vi "CZE20170723.vi"() -> ()   [LabVIEW 2016]
doc: "DESCRIPTION:\nThis VI simultaneously acquires and generates data on the same board (E-series MIO boards such as the AT-MIO-16E-2). This is a timed signal generation/acquisition, meaning that a hardware clock is used to control the acquisition and update rate for fast and accurate timing. While the output regenerates the same buffer of data, the input is a circular buffered acquisition. This means that a software buffer is used between your DAQ board and LabVIEW. While data is being transferred from your board into one part of the input buffer, LabVIEW is reading data from another part of that buffer. For this reason it is important that you set your acquisition parameters such that LabVIEW reads data out of the buffer fast enough to keep up with the rate at which your board is writing new data into the buffer. If not, unread data will be overwritten and an error will occur.\n\nDue to the fact that E-series MIO type boards have separate clocks dedicated to analog input and analog output, the acquisition and generation can occur at different rates. This example does not synchronize the two clocks.\n\nThis example does synchronize the start of the acquisition and generation using a software trigger. This is accomplished with AO Trigger and Gate Config (an advanced VI) with a trigger source set to \"AI Start Trigger\", which is a signal that will be generated internally when the acquisition begins. No external wiring is required. \n\nINSTRUCTIONS:\n1. Enter the device number, input channels, number of scans to read at a time, scan rate, and input buffer size.\n2. Enter the output channel, the update rate, the output buffer size, and choose the signal to output.\n3. Make the appropriate I/O connections as explained below.\n4. Run the VI.\n\nKEY PARAMETERS:\nThis VI shows how to use the intermediate analog input and analog output DAQ VIs to simultaneously input and output buffered data. On the diagram, notice that AO Start.vi is called before AI Start.vi due to the data dependency of the error cluster. This data dependency causes the acquisition to start after the generation has started.\n\nOn the diagram, notice that the AI Start.vi has a 0 wired for the number of scans to acquire, and the AO Start.vi has a 0 wired for the number of buffer iterations. This sets up continuous acquisition and generation.\n\nThis VI will try to use two DMA channels. If you do not have two available, you can use the Set DAQ Device Information.vi to set the data transfer mode for analog output and/or analog input to use interrupts. \n\nI/O CONNECTIONS:\nConnect to the output and input channels on the I/O connector for your board to match the channels you have chosen on the front panel of this VI.\n\nTo find the actual pin numbers, refer to your hardware user manual.\n\nDAQ VIs USED:\nAI Config.vi, AI Start.vi, AI Read.vi, AI Clear.vi, AO Config.vi, AO Write.vi, AO Trigger and Gate Config.vi, AO Start.vi, AO Clear.vi."
uses:
  <vilib>/Utility/error.llb/DialogType.ctl
  <vilib>/DAQmx/write.llb/DAQmx Write (Analog 1D DBL 1Chan NSamp).vi
  <vilib>/DAQmx/read.llb/DAQmx Read (Analog 2D DBL NChan NSamp).vi
  <vilib>/DAQmx/create/channels.llb/DAQmx Create Channel (AI-Voltage-Basic).vi
  <vilib>/DAQmx/configure/timing.llb/DAQmx Timing (Sample Clock).vi
  <vilib>/DAQmx/create/channels.llb/DAQmx Create Channel (AO-Voltage-Basic).vi
  <vilib>/DAQmx/configure/trigger.llb/DAQmx Start Trigger (Digital Edge).vi
  <vilib>/DAQmx/miscellaneous.llb/DAQmx Fill In Error Info.vi
  <vilib>/Utility/file.llb/Read From Spreadsheet File (DBL).vi
  <resource>/objmgr/daqmx.rc
panel:
  in  "DeviceName":tag="Dev2"
  in  "ケース定数\\n（詳細ヘルプを参照）":bool=TRUE
  in  "DC Volts":dbl=1200.0 min=-10000.0 max=10000.0 step=100.0
  in  "Wfm Type":bool=TRUE
  in  "Abort Load":bool
  in  "HIGH V ON":bool
  out "Time Remaining (sec)":dbl=-6.38378239159465e-16 format="%.1f"
  in  "Load Time (sec)":dbl=2.0 min=0.0 max=10000.0 step=10.0 format="%.1f"
  in  "Load Voltage":dbl=1200.0 min=0.0 max=100000.0 step=100.0
  in  "Load":bool
  out "Num Points":i32=180000
  in  "Duration (min)":dbl=300.0 min=0.0 step=1.0 format="%.1f"
  out "Period (sec)":dbl=0.10000000149011612 format="%.3f"
  in  "Pts/sec":sgl=10.0 min=0 max=10000 step=1 format="%.1f"
  out "Wfm Rate (Hz)":dbl=5.0 format="%.2f"
  out "REV/FWD":dbl=1.0 format="%.2f"
  out "FWD/REV":dbl=1.0 format="%.2f"
  in  "High V/V":dbl=1000.0 min=0.01 max=10000.0 step=100.0 format="%.2f"
  in  "REV Volts":dbl=-200.0 min=-10000.0 max=10000.0 step=100.0
  in  "REV Time (msec)":u32=100 min=1 max=100000 step=1
  in  "FWD Volts":dbl=200.0 min=-10000.0 max=10000.0 step=100.0
  in  "FWD Time (msec)":u32=100 min=1 max=100000 step=1
  out "file name":string
  in  "Read Data":bool
  in  "Start CZE":bool
  in  "Save Data":bool
  out "CZE":cluster{dbl[], dbl[]}(graph)={[0.0, 0.0016666666666666668, 0.0033333333333333335, 0.005, 0.006666666666666667, 0.008333333333333333, 0.01, 0.011666666666666667, 0.013333333333333334, 0.015000000000000001, 0.016666666666666666, 0.018333333333333333, 0.02, 0.021666666666666667, 0.023333333333333334, 0.025, 0.02666666666666667], [0.3002893448067642, 0.29141117530211785, 0.2338674873196842, 0.24110155064381295, 0.1523198704422416, 0.1661303531694248, 0.21249411892116374, 0.21413822415540437, 0.15922511176653875, 0.09674912167511775, 0.12141069594983661, 0.1046408253355316, 0.12864475792492638, 0.11878012798006383, 0.0845827453961778, 0.0655111290069393, 0.07800632588546134]} caption="CV"
  out "timed out?":bool
  in  "stop":bool
  # "DC"
  # "AC"
  # "S\nI\nG\nN\nA\nL\n\nV"
  # "TIME (min)"
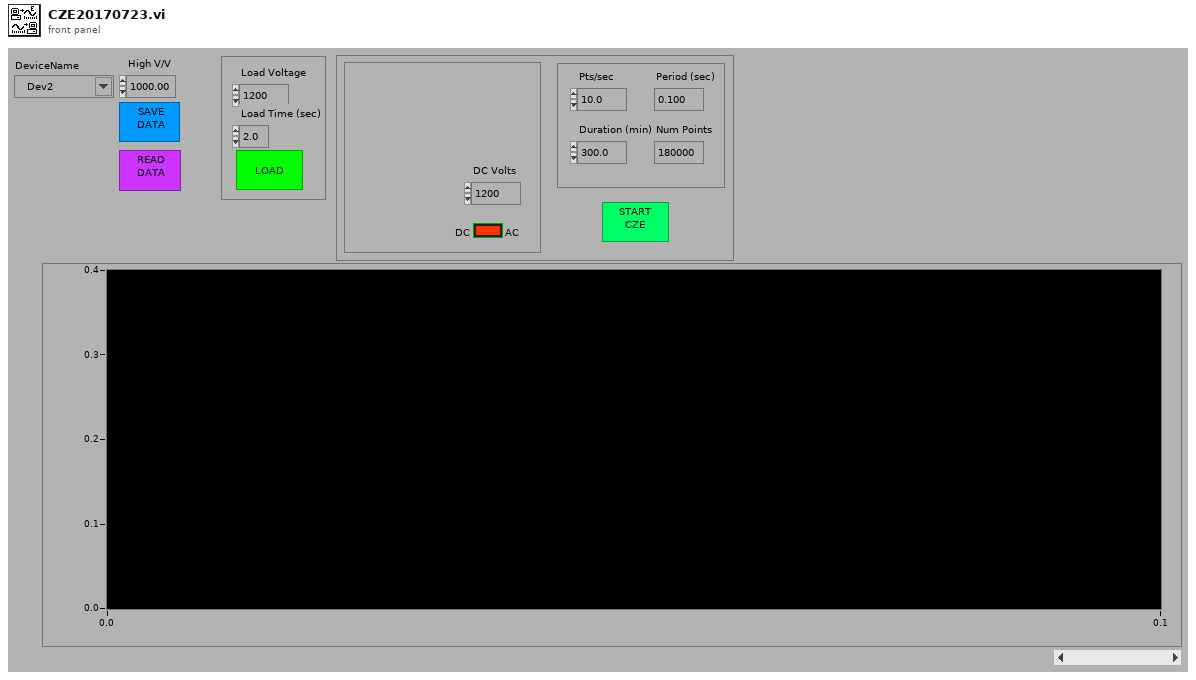
[diagram p1: front panel]
types:
  T1 = cluster{"high limit (0.0)":sgl, "low limit (0.0)":sgl}[]
  T2 = cluster{"coupling (no change:0)":enum16{"no change", "DC", "AC", "GND", "internal ref."}, "input config (no change:0)":enum16{"no change", "differential", "ref. single-ended", "non-ref. single-ended"}}[]
  T3 = enum16{"no change", "none", "trigger on rising edge", "trigger on falling edge", "pause while gate is TTL high", "pause while gate is TTL low"}
  T4 = enum16{"open", "open or create", "create or replace", "create"}
  T5 = typedef "DialogType.ctl" = u16
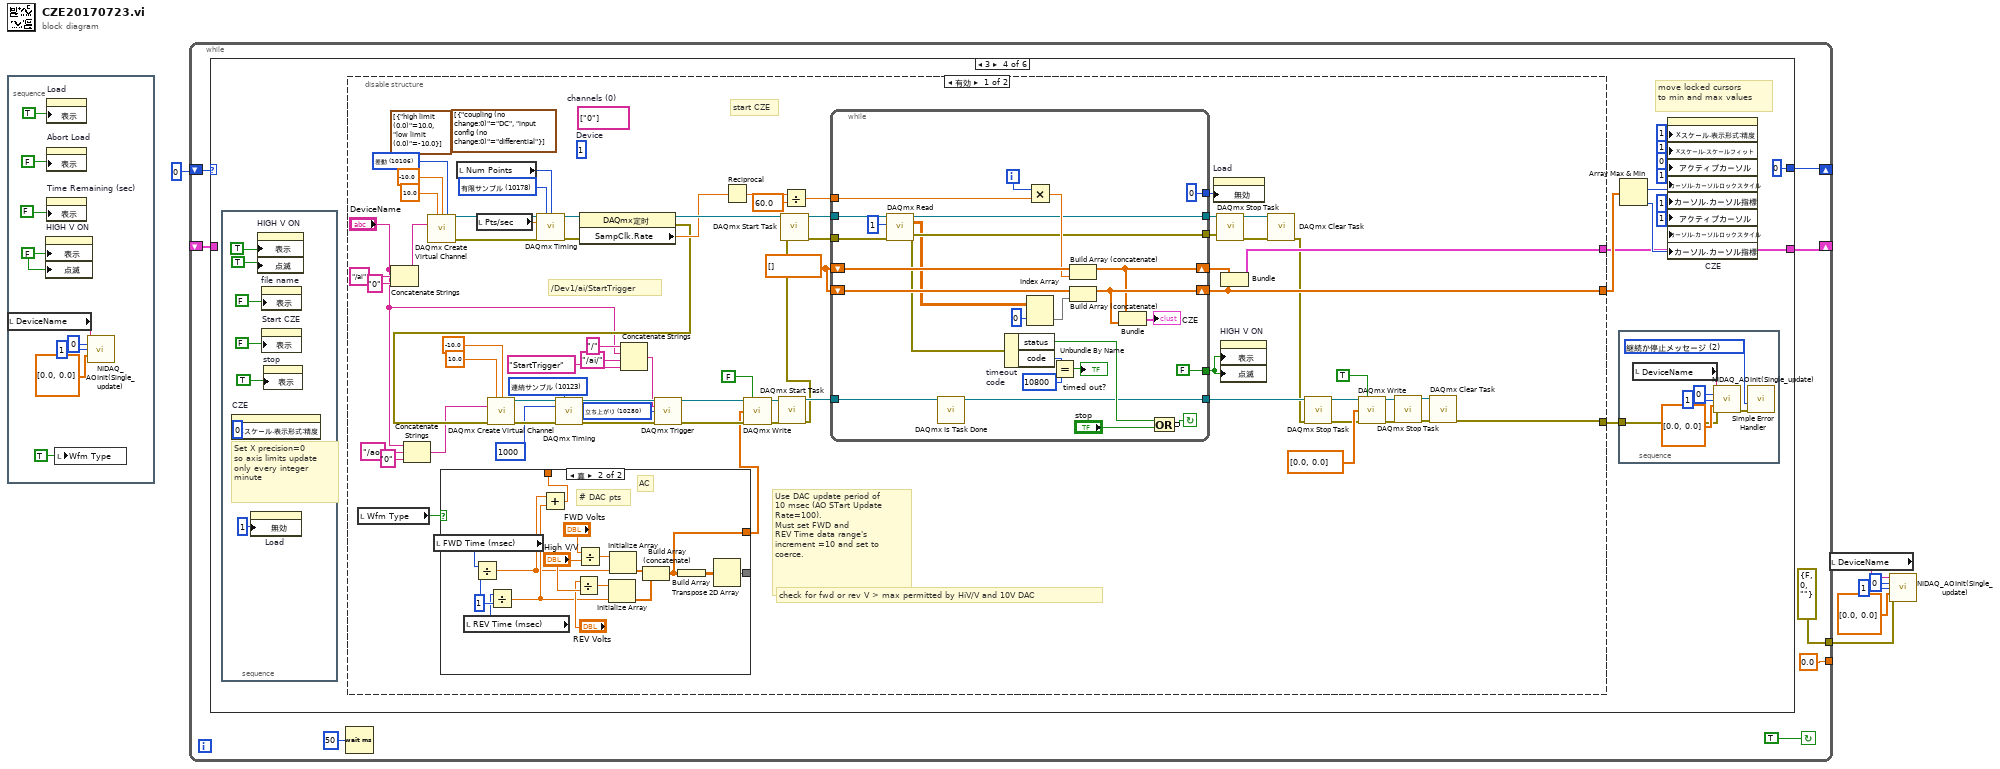
[diagram p0: block diagram]
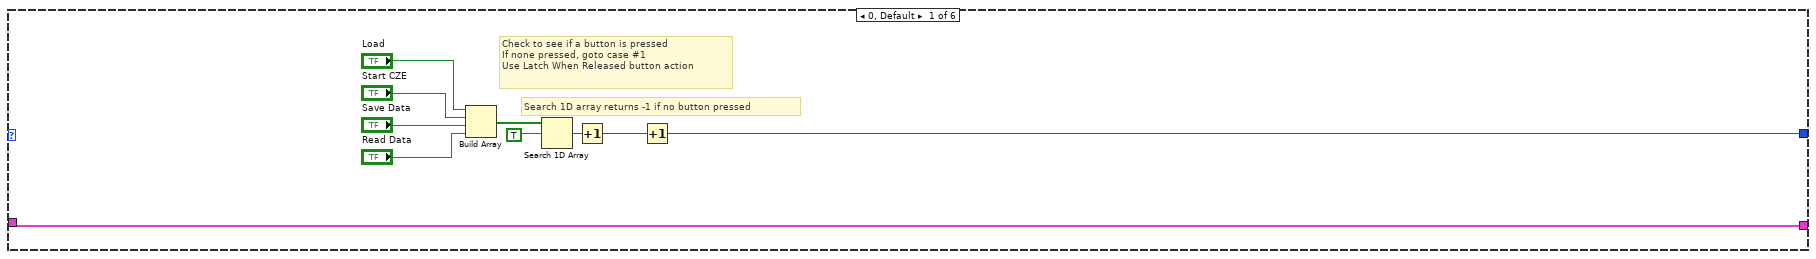
[diagram p2: hidden frame]
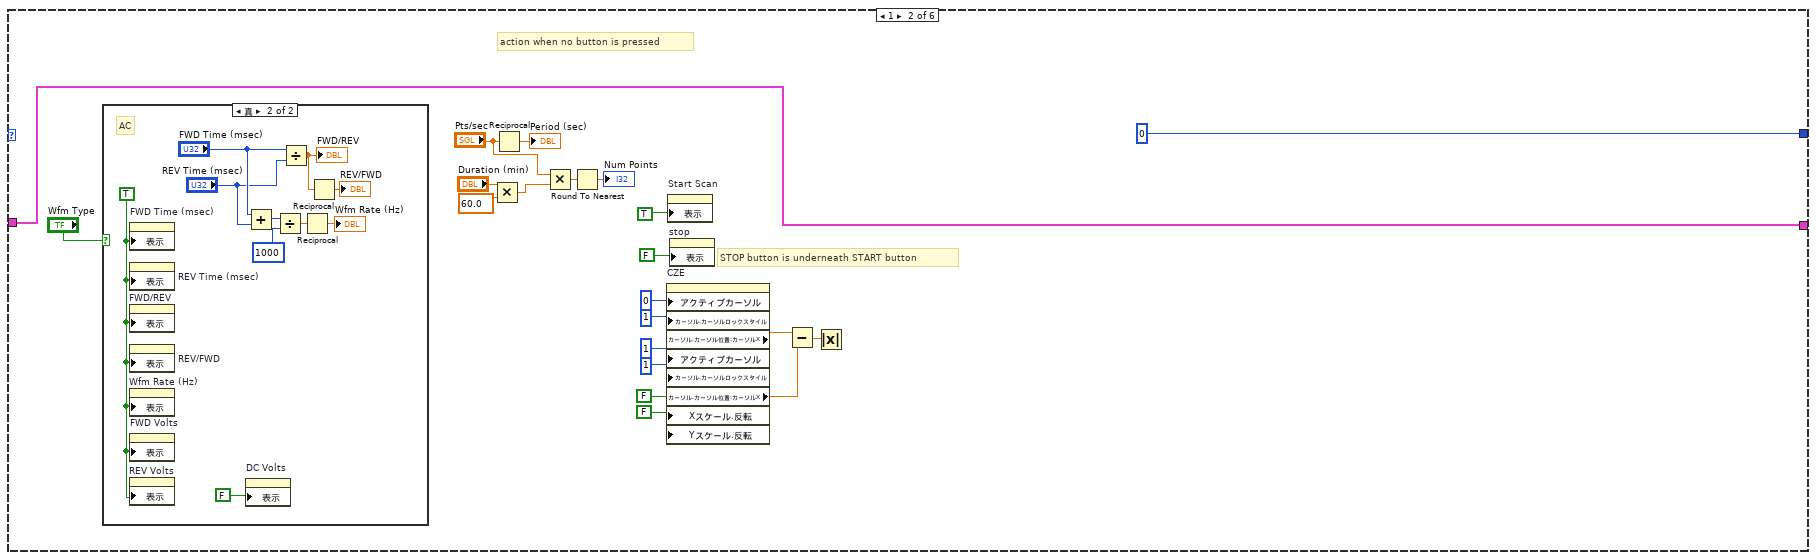
[diagram p3: hidden frame]
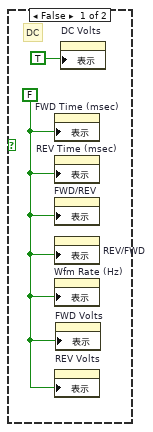
[diagram p4: hidden frame]
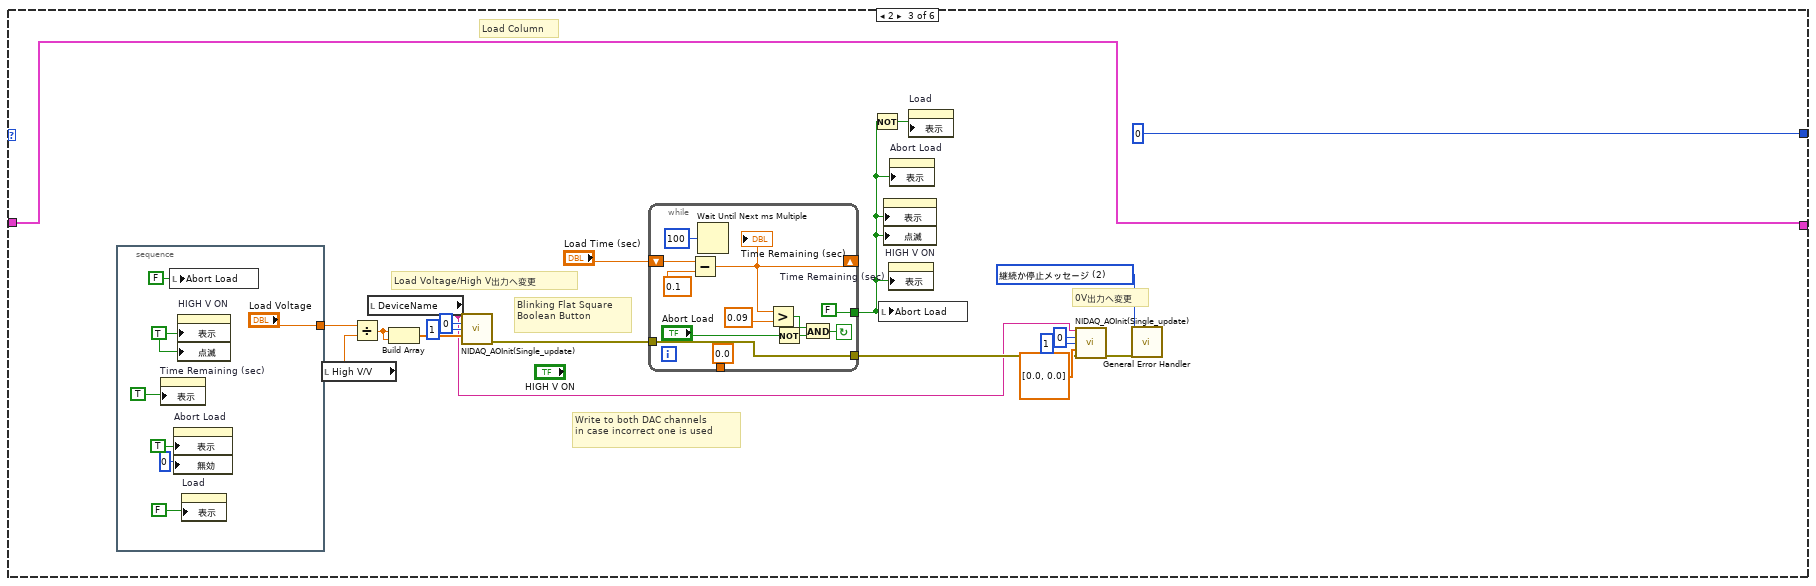
[diagram p5: hidden frame]
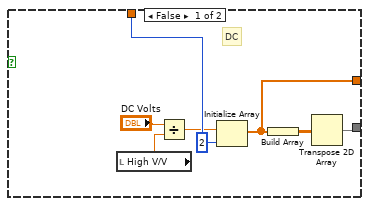
[diagram p6: hidden frame]
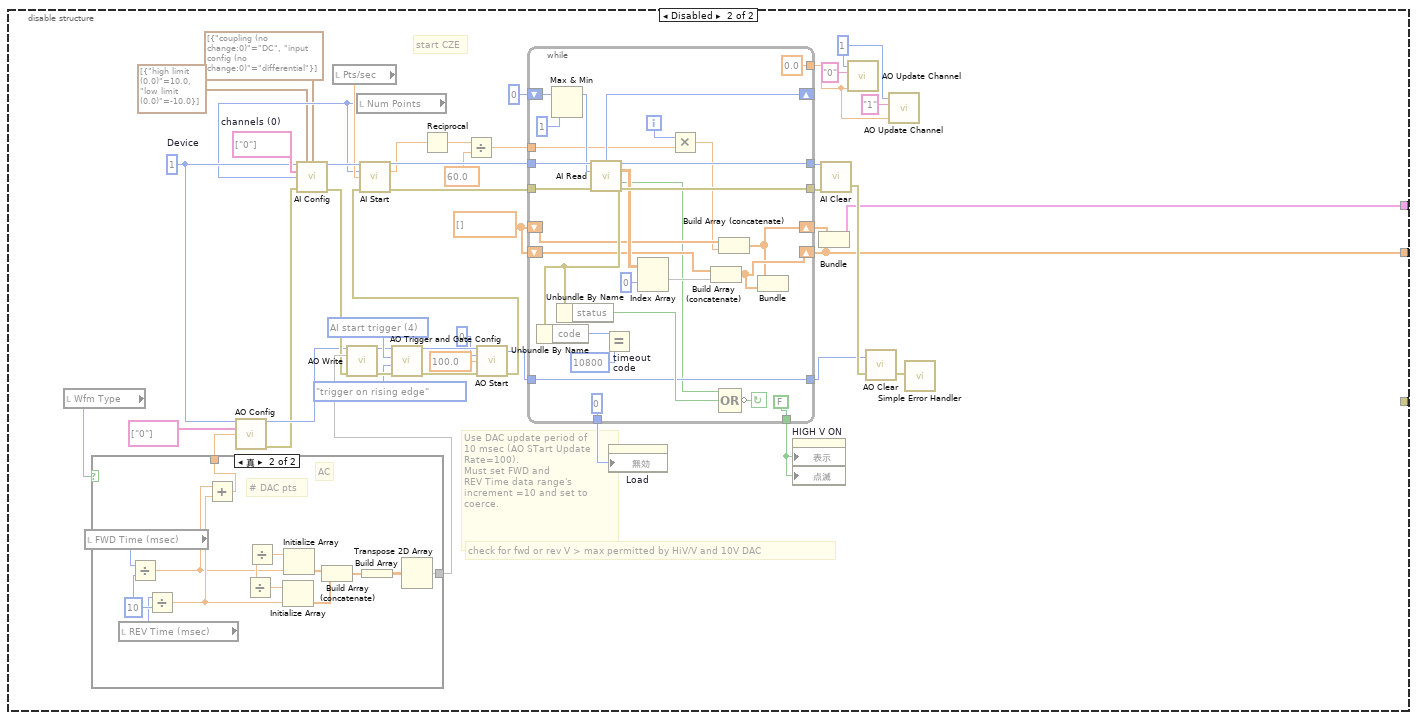
[diagram p7: hidden frame]
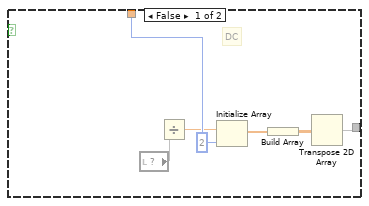
[diagram p8: hidden frame]
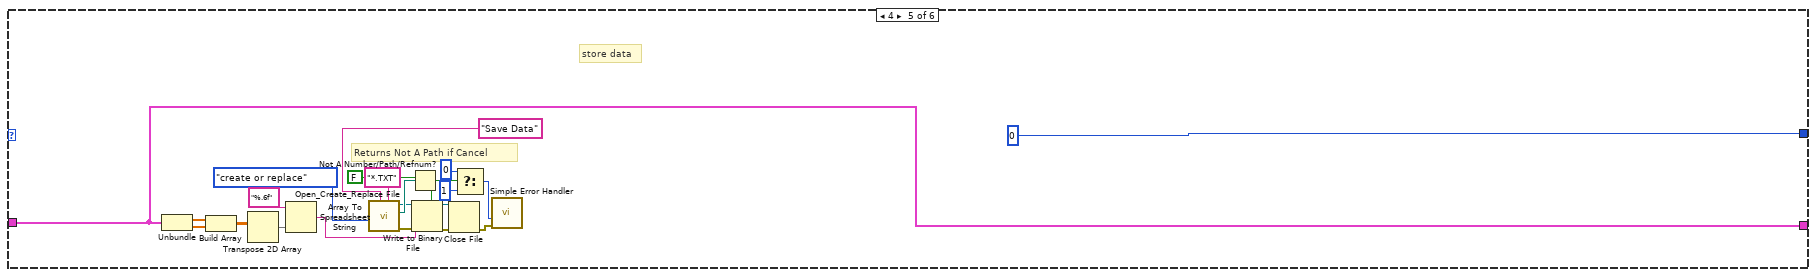
[diagram p9: hidden frame]
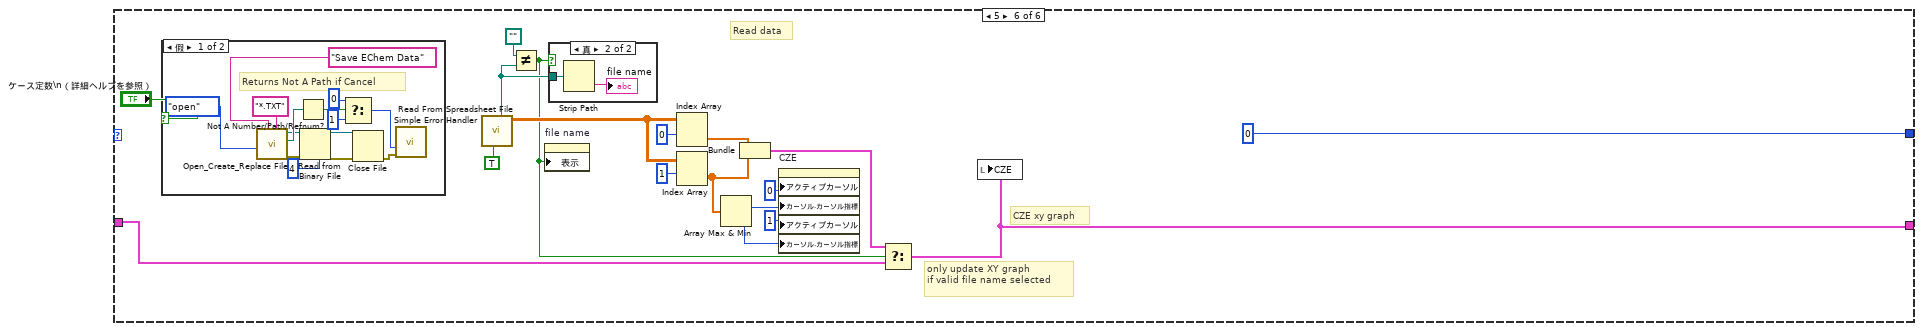
[diagram p10: hidden frame]
diagram:
  n1 = stacked-sequence {
    frame #0 {
      w13 = FALSE ("Visible")
      n2 = local read "DeviceName"() -> (w7:tag)
      n3 = property on="HIGH V ON" class="Bool"("表示"=w13, "点滅"=w13) -> ()  [unwired: 2 in, 2 out]
      n4 = property on="Load" class="Bool"("表示"=TRUE ("Visible")) -> ()  [unwired: 2 in, 2 out]
      n5 = property on="Abort Load" class="Bool (严格)"("表示"=FALSE ("Visible")) -> ()  [unwired: 2 in, 2 out]
      n6 = property on="Time Remaining (sec)" class="DigNum (严格)"("表示"=FALSE ("Visible")) -> ()  [unwired: 2 in, 2 out]
      n7 = local write "Wfm Type"(TRUE ("Wfm Type")) -> ()
      n8 = call "NIDAQ_AOInit(Single_update).vi"("DeviceName"=w7, "CH_A"=0, "CH_B"=1, "Single_point"=dbl[] [0.0, 0.0]) -> ()  [unwired: 11 in, 1 out]
    }
  }
  n9 = while {
    tunnel: [0.0] -> _
    shift-left: _ -> [w20]
    shift-right: [w21] -> _
    shift-left: 0 -> [w23]
    shift-right: [w22] -> _
    tunnel: [errorcluster {"status"=FALSE, "code"=0, "source"=""} ("error in (no error)")] -> w2
    stop <- TRUE continue-if-true
    n10 = case shown="3" w23 {
      tunnel: [w25 0 0 ("t") 0 0 0 ("t")] -> w22
      tunnel: [w28 w44 w83 w108 w348 w368] -> w21
      tunnel: w20 -> [w28 w44 w83 _ w348 w366]
      frame 0, Default {
        # "Check to see if a button is pressed\nIf none pressed, goto case #1\nUse Latch When Released button action"
        # "Search 1D array returns -1 if no button pressed"
        n11 = Build Array("Load", "Start CZE", "Save Data", "Read Data") -> (w31:bool[])
        n12 = Search 1D Array(1D array=w31, element=TRUE) -> (index of element=w29:i32)  [unwired: 1 in]
        n13 = Increment(x=w29) -> (x+1=w27:i32)
        n14 = Increment(x=w27) -> (x+1=w25:i32)
      }
      frame 1 {
        # "STOP button is underneath START button"
        # "action when no button is pressed"
        n15 = case shown="真" "Wfm Type" {
          frame False {
            w55 = FALSE
            # "DC"
            n16 = property on="FWD Time (msec)" class="DigNum (严格)"("表示"=w55) -> ()  [unwired: 2 in, 2 out]
            n17 = property on="REV Time (msec)" class="DigNum (严格)"("表示"=w55) -> ()  [unwired: 2 in, 2 out]
            n18 = property on="FWD/REV" class="DigNum (严格)"("表示"=w55) -> ()  [unwired: 2 in, 2 out]
            n19 = property on="REV/FWD" class="DigNum (严格)"("表示"=w55) -> ()  [unwired: 2 in, 2 out]
            n20 = property on="Wfm Rate (Hz)" class="DigNum (严格)"("表示"=w55) -> ()  [unwired: 2 in, 2 out]
            n21 = property on="REV Volts" class="DigNum (严格)"("表示"=w55) -> ()  [unwired: 2 in, 2 out]
            n22 = property on="FWD Volts" class="DigNum (严格)"("表示"=w55) -> ()  [unwired: 2 in, 2 out]
            n23 = property on="DC Volts" class="DigNum (严格)"("表示"=TRUE ("Visible")) -> ()  [unwired: 2 in, 2 out]
          }
          frame True {
            w58 = TRUE
            # "AC"
            n24 = property on="FWD Time (msec)" class="DigNum (严格)"("表示"=w58) -> ()  [unwired: 2 in, 2 out]
            n25 = property on="REV Time (msec)" class="DigNum (严格)"("表示"=w58) -> ()  [unwired: 2 in, 2 out]
            n26 = property on="FWD/REV" class="DigNum (严格)"("表示"=w58) -> ()  [unwired: 2 in, 2 out]
            n27 = property on="REV/FWD" class="DigNum (严格)"("表示"=w58) -> ()  [unwired: 2 in, 2 out]
            n28 = property on="Wfm Rate (Hz)" class="DigNum (严格)"("表示"=w58) -> ()  [unwired: 2 in, 2 out]
            n29 = property on="FWD Volts" class="DigNum (严格)"("表示"=w58) -> ()  [unwired: 2 in, 2 out]
            n30 = property on="REV Volts" class="DigNum (严格)"("表示"=w58) -> ()  [unwired: 2 in, 2 out]
            n31 = Add(x="FWD Time (msec)", y="REV Time (msec)") -> (x+y=w64:u32)
            n32 = property on="DC Volts" class="DigNum (严格)"("表示"=FALSE ("Visible")) -> ()  [unwired: 2 in, 2 out]
            n33 = Divide(x=w64, y=u32 1000) -> (x/y=w60:dbl)
            n34 = Divide(x="FWD Time (msec)", y="REV Time (msec)") -> (x/y=w66:dbl)
            "FWD/REV" <- w66
            n35 = Reciprocal(x=w60) -> (1/x=→"Wfm Rate (Hz)":dbl)
            n36 = Reciprocal(x=w66) -> (1/x=→"REV/FWD":dbl)
          }
        }
        n37 = Multiply(x="Duration (min)", y=60.0) -> (x*y=w38:dbl)
        n38 = Reciprocal(x="Pts/sec") -> (1/x=→"Period (sec)":sgl)
        n39 = Multiply(x="Pts/sec", y=w38) -> (x*y=w41:dbl)
        n40 = Round To Nearest(number=w41) -> (nearest integer value=→"Num Points":dbl)
        n41 = property on="CZE" class="XYGraph (严格)"("アクティブカーソル"=u32 0 ("Active Cursor"), "カーソル.カーソルロックスタイル"=u32 1 ("Cursor Locked"), "アクティブカーソル"=u32 1 ("Active Cursor"), "カーソル.カーソルロックスタイル"=u32 1 ("Cursor Locked"), "Xスケール.反転"=FALSE ("X Flipped"), "Yスケール.反転"=FALSE ("Y Flipped")) -> ("カーソル.カーソル位置:カーソルX"=w48:dbl, "カーソル.カーソル位置:カーソルX"=w47:dbl)  [unwired: 2 in, 2 out]
        n42 = property on="Start Scan" class="Bool"("表示"=TRUE ("Visible")) -> ()  [unwired: 2 in, 2 out]
        n43 = property on="stop" class="Bool"("表示"=FALSE ("Visible")) -> ()  [unwired: 2 in, 2 out]
        n44 = Subtract(x=w48, y=w47) -> (x-y=w49:dbl)
        n45 = Absolute Value(x=w49) -> ()  [unwired: 1 out]
      }
      frame 2 {
        w67 = T5 2 items=["ダイアログなし", "OKメッセージ", "継続か停止メッセージ", "OKメッセージ+警告", "継続/停止+警告"] ("type of dialog (OK msg:1)")
        # "Load Voltage/High V出力へ変更"
        # "0V出力へ変更"
        # "Blinking Flat Square\nBoolean Button"
        # "Write to both DAC channels\nin case incorrect one is used"
        # "Load Column"
        n46 = stacked-sequence {
          tunnel: ["Load Voltage"] -> w82
          frame #0 {
            w104 = TRUE ("Visible")
            n47 = property on="Time Remaining (sec)" class="DigNum (严格)"("表示"=TRUE ("Visible")) -> ()  [unwired: 2 in, 2 out]
            n48 = local write "Abort Load"(FALSE ("Abort Load")) -> ()
            n49 = property on="Abort Load" class="Bool (严格)"("表示"=TRUE ("Visible"), "無効"=u8 0 ("Disabled")) -> ()  [unwired: 2 in, 2 out]
            n50 = property on="HIGH V ON" class="Bool"("表示"=w104, "点滅"=w104) -> ()  [unwired: 2 in, 2 out]
            n51 = property on="Load" class="Bool"("表示"=FALSE ("Visible")) -> ()  [unwired: 2 in, 2 out]
          }
        }
        n52 = local read "High V/V"() -> (w81:dbl)
        n53 = Divide(x=w82, y=w81) -> (x/y=w73:dbl)
        n54 = local read "DeviceName"() -> (w69:tag)
        n55 = Build Array(w73, w73) -> (w72:dbl[])
        n56 = call "NIDAQ_AOInit(Single_update).vi"("DeviceName"=w69, "CH_A"=0, "CH_B"=1, "Single_point"=w72) -> ("error out"=w71:errorcluster)  [unwired: 11 in]
        n57 = while {
          tunnel: [0.0] -> _
          tunnel: [FALSE] -> w79
          shift-left: "Load Time (sec)" -> [w96]
          shift-right: [w87] -> _
          tunnel: w71 -> [w86]
          tunnel: [w86] -> w70
          stop <- w94 continue-if-true
          n58 = Subtract(x=w96, y=0.1) -> (x-y=w87:dbl)
          "Time Remaining (sec)" <- w87
          n59 = Wait Until Next ms Multiple(millisecond multiple=u32 100) -> ()  [unwired: 1 out]
          n60 = Greater?(x=w87, y=0.09) -> (0:w93:bool)
          n61 = Not(x="Abort Load") -> (.not. x?=w91:bool)
          n62 = And(x=w93, y=w91) -> (x .and. y?=w94:bool)
        }
        n63 = Not(x=w79) -> (.not. x?=w84:bool)
        n64 = local write "Abort Load"(w79) -> ()
        n65 = property on="HIGH V ON" class="Bool"("表示"=w79, "点滅"=w79) -> ()  [unwired: 2 in, 2 out]
        n66 = property on="Time Remaining (sec)" class="DigNum (严格)"("表示"=w79) -> ()  [unwired: 2 in, 2 out]
        n67 = property on="Abort Load" class="Bool (严格)"("表示"=w79) -> ()  [unwired: 2 in, 2 out]
        n68 = property on="Load" class="Bool"("表示"=w84) -> ()  [unwired: 2 in, 2 out]
        n69 = call "NIDAQ_AOInit(Single_update).vi"("DeviceName"=w69, "CH_A"=0, "CH_B"=1, "Single_point"=dbl[] [0.0, 0.0], "error in (no error)"=w70) -> ("error out"=w68:errorcluster)  [unwired: 10 in]
        n70 = call <vilib>:"General Error Handler.vi"("type of dialog (OK msg:1)"=w67, "error in (no error)"=w68) -> ()  [unwired: 9 in, 5 out]
      }
      frame 3 {
        # "move locked cursors\nto min and max values"
        n71 = stacked-sequence {
          frame #0 {
            # "Set X precision=0\nso axis limits update\nonly every integer\nminute"
            n72 = property on="CZE" class="XYGraph (严格)"("Xスケール.表示形式:精度"=u8 0 ("X Precision")) -> ()  [unwired: 2 in, 2 out]
            n73 = property on="Load" class="Bool"("無効"=u8 1 ("Disabled")) -> ()  [unwired: 2 in, 2 out]
            n74 = property on="HIGH V ON" class="Bool"("表示"=TRUE ("Visible"), "点滅"=TRUE ("Blinking")) -> ()  [unwired: 2 in, 2 out]
            n75 = property on="file name" class="Str"("表示"=FALSE ("Visible")) -> ()  [unwired: 2 in, 2 out]
            n76 = property on="Start CZE" class="Bool"("表示"=FALSE ("Visible")) -> ()  [unwired: 2 in, 2 out]
            n77 = property on="stop" class="Bool"("表示"=TRUE ("Visible")) -> ()  [unwired: 2 in, 2 out]
          }
        }
        n78 = disable-structure shown="有効" {
          disable-tunnel: [w191 w263] -> w113
          disable-tunnel: [w189 w261] -> w108
          disable-tunnel: [w126 _] -> w105
          frame Enabled {
            w161 = 10178 items=["有限サンプル"=10178, "連続サンプル"=10123, "ハードウェアタイミングシングルポイント"=12522] ("sample mode")
            w169 = 10106 items=["デフォルト"=-1, "基準化シングルエンド"=10083, "非基準化シングルエンド"=10078, "差動"=10106, "擬似差動"=12529] ("input terminal configuration")
            w170 = 10123 items=["有限サンプル"=10178, "連続サンプル"=10123, "ハードウェアタイミングシングルポイント"=12522] ("sample mode")
            w180 = 10280 items=["立ち上がり"=10280, "立ち下がり"=10171] ("edge")
            (unwired) T1 [{"high limit (0.0)"=10.0, "low limit (0.0)"=-10.0}] ("input limits (no change)")
            (unwired) T2 [{"coupling (no change:0)"=enum."DC", "input config (no change:0)"=enum."differential"}] ("coupling & input config (no change:0)")
            (unwired) i16 1  # Device
            (unwired) string[] ["0"]  # channels (0)
            w188 = sgl[] []
            # "/Dev1/ai/StartTrigger"
            # "Use DAC update period of\n10 msec (AO STart Update\nRate=100).\nMust set FWD and\nREV Time data range's\nincrement =10 and set to\ncoerce."
            # "check for fwd or rev V > max permitted by HiV/V and 10V DAC"
            # "start CZE"
            n79 = local read "Wfm Type"() -> (w182:bool)
            n80 = Concatenate Strings("DeviceName", "/ai", "0" ("文字列")) -> (w147:string)
            n81 = Concatenate Strings("DeviceName", "/ao", "0" ("文字列")) -> (w144:string)
            n82 = call-poly <vilib>:"DAQmx Create Virtual Channel.vi"("maximum value"=10.0, "minimum value"=-10.0, "input terminal configuration"=w169, "physical channels"=w147) -> ("task out"=w156:refnum<k21>, "error out"=w164:errorcluster)  [unwired: 10 in]
            n83 = case shown="真" w182 {
              tunnel: [w224 w240] -> _
              tunnel: [w222 w226] -> _
              tunnel: [w218 w225] -> w135
              frame False {
                w222 = 2
                # "DC"
                n84 = local read "High V/V"() -> (w219:dbl)
                n85 = Divide(x="DC Volts", y=w219) -> (x/y=w221:dbl)
                n86 = Initialize Array(w221, w222) -> (w218:dbl[])
                n87 = Build Array(w218) -> (w223:dbl[][])
                n88 = Transpose 2D Array(2D array=w223) -> (transposed array=w224:dbl[][])
              }
              frame True {
                w234 = u32 1 ("y")
                # "AC"
                # "# DAC pts"
                n89 = local read "FWD Time (msec)"() -> (w232:u32)
                n90 = local read "REV Time (msec)"() -> (w233:u32)
                n91 = Divide(x=w232, y=w234) -> (x/y=w227:dbl)
                n92 = Divide(x=w233, y=w234) -> (x/y=w228:dbl)
                n93 = Add(x=w227, y=w228) -> (x+y=w226:dbl)
                n94 = Divide(x="REV Volts", y="High V/V") -> (x/y=w236:dbl)
                n95 = Divide(x="FWD Volts", y="High V/V") -> (x/y=w237:dbl)
                n96 = Initialize Array(w236, w228) -> (w230:dbl[])
                n97 = Initialize Array(w237, w227) -> (w231:dbl[])
                n98 = Build Array (concatenate)(w231, w230) -> (w225:dbl[])
                n99 = Build Array(w225) -> (w229:dbl[][])
                n100 = Transpose 2D Array(2D array=w229) -> (transposed array=w240:dbl[][])
              }
            }
            n101 = local read "Num Points"() -> (w162:i32)
            n102 = local read "Pts/sec"() -> (w163:sgl)
            n103 = call-poly <vilib>:"DAQmx Timing.vi"("task/channels in"=w156, "sample mode"=w161, "samples per channel"=w162, "rate"=w163, "error in"=w164) -> ("task out"=w160:refnum<k21>, "error out"=w159:errorcluster)  [unwired: 9 in]
            n104 = property class="DAQmx定时"(reference=w160, error in=w159) -> (reference out=w158:refnum<k21>, error out=w154:errorcluster, "SampClk.Rate"=w157:dbl)
            n105 = call-poly <vilib>:"DAQmx Create Virtual Channel.vi"("maximum value"=10.0, "minimum value"=-10.0, "physical channels"=w144, "error in"=w154) -> ("task out"=w174:refnum<k21>, "error out"=w171:errorcluster)  [unwired: 10 in]
            n106 = call-poly <vilib>:"DAQmx Timing.vi"("task/channels in"=w174, "sample mode"=w170, "rate"=1000, "error in"=w171) -> ("task out"=w173:refnum<k21>, "error out"=w172:errorcluster)  [unwired: 10 in]
            n107 = Concatenate Strings("/", "DeviceName", "/ai/", "StartTrigger" ("文字列")) -> (w140:string)
            n108 = call-poly <vilib>:"DAQmx Trigger.vi"("task/channels in"=w173, "source"=w140, "edge"=w180, "error in"=w172) -> ("task out"=w139:refnum<k21>, "error out"=w138:errorcluster)  [unwired: 10 in]
            n109 = Reciprocal(x=w157) -> (1/x=w185:dbl)
            n110 = call-poly <vilib>:"DAQmx Write.vi"("task/channels in"=w139, "auto start"=FALSE, "data"=w135, "error in"=w138) -> ("task out"=w179:refnum<k21>, "error out"=w178:errorcluster)  [unwired: 9 in, 1 out]
            n111 = call <vilib>:"DAQmx Start Task.vi"("task/channels in"=w179, "error in"=w178) -> ("task out"=w177:refnum<k21>, "error out"=w153:errorcluster)  [unwired: 12 in]
            n112 = call <vilib>:"DAQmx Start Task.vi"("task/channels in"=w158, "error in"=w153) -> ("task out"=w152:refnum<k21>, "error out"=w155:errorcluster)  [unwired: 12 in]
            n113 = Divide(x=w185, y=sgl 60.0) -> (x/y=w187:dbl)
            n114 = while {
              tunnel: [u8 0] -> w183
              tunnel: [FALSE] -> w184
              tunnel: w187 -> [w205]
              shift-left: w188 -> [w211]
              shift-right: [w210] -> w191
              shift-left: w188 -> [w212]
              shift-right: [w206] -> w190
              tunnel: [w197] -> w150
              tunnel: [w199] -> w137
              tunnel: w177 -> [w198]
              tunnel: w155 -> [w196]
              tunnel: w152 -> [w195]
              tunnel: [w194] -> w151
              i -> [w204]
              stop <- w217 continue-if-true
              w215 = 10800  # timeout code
              n115 = call-poly <vilib>:"DAQmx Read.vi"("task/channels in"=w195, "number of samples per channel"=1, "error in"=w196) -> ("task out"=w194:refnum<k21>, "data"=w193:dbl[][], "error out"=w197:errorcluster)  [unwired: 10 in]
              n116 = call <vilib>:"DAQmx Is Task Done.vi"("task/channels in"=w198) -> ("task out"=w199:refnum<k21>)  [unwired: 12 in, 2 out]
              n117 = Unbundle By Name(w197) -> ("status"=w216:bool, "code"=w200:i32)
              n118 = Multiply(x=w204, y=w205) -> (x*y=w203:dbl)
              n119 = Index Array(array=w193, index (col)=0) -> (element=w207:dbl[])  [unwired: 1 in]
              n120 = Equal?(x=w200, y=w215) -> (x = y?=→"timed out?":bool)
              n121 = Build Array (concatenate)(w212, w203) -> (w206:dbl[])
              n122 = Build Array (concatenate)(w211, w207) -> (w210:dbl[])
              n123 = Bundle(w206, w210) -> (→"CZE":cluster{dbl[], dbl[]})  [unwired: 1 in]
              n124 = Compound Arithmetic op=OR(w216, "stop") -> (invert w217:bool)
            }
            n125 = property on="Load" class="Bool"("無効"=w183) -> ()  [unwired: 2 in, 2 out]
            n126 = call <vilib>:"DAQmx Stop Task.vi"("task/channels in"=w151, "error in"=w150) -> ("task out"=w166:refnum<k21>, "error out"=w165:errorcluster)  [unwired: 12 in]
            n127 = property on="HIGH V ON" class="Bool"("表示"=w184, "点滅"=w184) -> ()  [unwired: 2 in, 2 out]
            n128 = Bundle(w190, w191) -> (w189:cluster{dbl[], dbl[]})  [unwired: 1 in]
            n129 = call <vilib>:"DAQmx Clear Task.vi"("task in"=w166, "error in"=w165) -> ("error out"=w136:errorcluster)  [unwired: 13 in]
            n130 = call <vilib>:"DAQmx Stop Task.vi"("task/channels in"=w137, "error in"=w136) -> ("task out"=w132:refnum<k21>, "error out"=w131:errorcluster)  [unwired: 12 in]
            n131 = call-poly <vilib>:"DAQmx Write.vi"("task/channels in"=w132, "auto start"=TRUE, "data"=dbl[] [0.0, 0.0], "error in"=w131) -> ("task out"=w130:refnum<k21>, "error out"=w129:errorcluster)  [unwired: 9 in, 1 out]
            n132 = call <vilib>:"DAQmx Stop Task.vi"("task/channels in"=w130, "error in"=w129) -> ("task out"=w128:refnum<k21>, "error out"=w127:errorcluster)  [unwired: 12 in]
            n133 = call <vilib>:"DAQmx Clear Task.vi"("task in"=w128, "error in"=w127) -> ("error out"=w126:errorcluster)  [unwired: 13 in]
          }
          frame Disabled {
            w254 = i16 1 ("device")
            w259 = i16 1  # Device
            w268 = string[] ["0"]  # channels (0)
            w249 = sgl[] []
            w276 = u16 4 items=["no change", "none", "PFI pin", "RTSI pin", "AI start trigger", "ATCOUT", "trigger input connector"] ("trigger or gate source (0: no change)")
            # "Use DAC update period of\n10 msec (AO STart Update\nRate=100).\nMust set FWD and\nREV Time data range's\nincrement =10 and set to\ncoerce."
            # "check for fwd or rev V > max permitted by HiV/V and 10V DAC"
            # "start CZE"
            n134 = local read "Wfm Type"() -> (w241:bool)
            n135 = case shown="真" w241 {
              tunnel: [w321 w336] -> w272
              tunnel: [w318 w322] -> w257
              frame False {
                w318 = 2
                # "DC"
                n136 = local read item#-1() -> (w316)
                n137 = Divide(y=w316) -> (x/y=w317:dbl)  [unwired: 1 in]
                n138 = Initialize Array(w317, w318) -> (w319:dbl[])
                n139 = Build Array(w319) -> (w320:dbl[][])
                n140 = Transpose 2D Array(2D array=w320) -> (transposed array=w321:dbl[][])
              }
              frame True {
                w331 = u32 10 ("y")
                # "AC"
                # "# DAC pts"
                n141 = local read "FWD Time (msec)"() -> (w329:u32)
                n142 = local read "REV Time (msec)"() -> (w330:u32)
                n143 = Divide(x=w329, y=w331) -> (x/y=w323:dbl)
                n144 = Divide(x=w330, y=w331) -> (x/y=w324:dbl)
                n145 = Add(x=w323, y=w324) -> (x+y=w322:dbl)
                n146 = Divide() -> (y=w335:dbl, x/y=w334:dbl)  [unwired: 1 in]
                n147 = Divide(y=w335) -> (x=w332:dbl, x/y=w333:dbl)
                n148 = Initialize Array(w333, w324) -> (w327:dbl[])
                n149 = Initialize Array(w334, w323) -> (w328:dbl[])
                n150 = Build Array (concatenate)(w328, w327) -> (w325:dbl[])
                n151 = Build Array(w325) -> (w326:dbl[][])
                n152 = Transpose 2D Array(2D array=w326) -> (transposed array=w336:dbl[][])
              }
            }
            n153 = call "AO Config.vi"("device (1)"=w259, "channels (0)"=string[] ["0"], "buffer size (1000 updates)"=w257) -> ("taskID"=w265:u32, "error out"=w264:errorcluster)  [unwired: 10 in, 1 out]
            n154 = local read "Pts/sec"() -> (w252:sgl)
            n155 = local read "Num Points"() -> (w251:i32)
            n156 = call "AI Config.vi"("device (1)"=w259, "input limits (no change)"=T1 [{"high limit (0.0)"=10.0, "low limit (0.0)"=-10.0}], "coupling & input config (no change:0)"=T2 [{"coupling (no change:0)"=enum."DC", "input config (no change:0)"=enum."differential"}], "channels (0)"=w268, "buffer size (1000 scans)"=w251, "error in (no error)"=w264) -> ("taskID"=w286:u32, "error out"=w266:errorcluster)  [unwired: 7 in, 1 out]
            n157 = call-poly "AO Write.vi"("taskID in"=w265, "scaled data"=w272, "error in (no error)"=w266) -> ("taskID out"=w275:u32, "error out"=w274:errorcluster)  [unwired: 8 in, 3 out]
            n158 = call "AO Trigger and Gate Config.vi"("error in (no error)"=w274, "trigger or gate condition (0: no change)"=T3."trigger on rising edge", "trigger or gate source (0: no change)"=w276, "task ID"=w275) -> ("error out"=w277:errorcluster, "task ID out"=w279:u32)  [unwired: 6 in]
            n159 = call "AO Start.vi"("taskID in"=w279, "number of buffer iterations (1)"=0, "update rate (1000 updates/sec)"=sgl 100.0, "error in (no error)"=w277) -> ("taskID out"=w270:u32, "error out"=w278:errorcluster)  [unwired: 9 in, 1 out]
            n160 = call "AI Start.vi"("taskID in"=w286, "number of scans to acquire (-1)"=w251, "scan rate (1000 scans/sec)"=w252, "error in (no error)"=w278) -> ("taskID out"=w285:u32, "actual scan rate"=w260:sgl, "error out"=w280:errorcluster)  [unwired: 8 in, 1 out]
            n161 = Reciprocal(x=w260) -> (1/x=w246:sgl)
            n162 = Divide(x=w246, y=sgl 60.0) -> (x/y=w248:sgl)
            n163 = while {
              tunnel: [u8 0] -> w242
              tunnel: [FALSE] -> w245
              tunnel: [0.0] -> w253
              tunnel: w248 -> [w292]
              shift-left: u32 0 ("scan backlog") -> [w301]
              shift-right: [w302] -> _
              shift-left: w249 -> [w304]
              shift-right: [w303] -> w263
              shift-left: w249 -> [w305]
              shift-right: [w293] -> w262
              tunnel: w280 -> [w311]
              tunnel: [w296] -> w271
              tunnel: w270 -> [w296]
              tunnel: w285 -> [w314]
              tunnel: [w315] -> w284
              tunnel: [w310] -> w283
              i -> [w291]
              stop <- w313 continue-if-true
              w309 = 10800  # timeout code
              n164 = Max & Min(x=w301, y=u32 1 ("x")) -> (max(x,y)=w299:u32)  [unwired: 1 out]
              n165 = call-poly "AI Read.vi"("taskID in"=w314, "number of scans to read (-1:all)"=w299, "error in (no error)"=w311) -> ("scan backlog"=w302:u32, "taskID out"=w315:u32, "scaled data"=w306:sgl[][], "retrieval complete"=w288:bool, "error out"=w310:errorcluster)  [unwired: 7 in, 1 out]
              n166 = Unbundle By Name(w310) -> ("code"=w308:i32)
              n167 = Unbundle By Name(w310) -> ("status"=w312:bool)
              n168 = Equal?(x=w308, y=w309) -> ()  [unwired: 1 out]
              n169 = Index Array(array=w306, index (col)=0) -> (element=w295:sgl[])  [unwired: 1 in]
              n170 = Multiply(x=w291, y=w292) -> (x*y=w290:sgl)
              n171 = Build Array (concatenate)(w304, w295) -> (w303:sgl[])
              n172 = Build Array (concatenate)(w305, w290) -> (w293:sgl[])
              n173 = Compound Arithmetic op=OR(w288, w312) -> (invert w313:bool, w298:bool)
              n174 = Bundle(w293, w303) -> (w297:cluster{sgl[], sgl[]})  [unwired: 1 in]
            }
            n175 = property on="Load" class="Bool"("無効"=w242) -> ()  [unwired: 2 in, 2 out]
            n176 = property on="HIGH V ON" class="Bool"("表示"=w245, "点滅"=w245) -> ()  [unwired: 2 in, 2 out]
            n177 = Bundle(w262, w263) -> (w261:cluster{sgl[], sgl[]})  [unwired: 1 in]
            n178 = call "AI Clear.vi"("error in (no error)"=w283, "taskID in"=w284) -> ("error out"=w281:errorcluster)  [unwired: 4 in, 1 out]
            n179 = call-poly "AO Update Channel.vi"("value"=w253, "channel (0)"="0", "device"=w254) -> ()
            n180 = call "AO Clear.vi"("error in (no error)"=w281, "taskID in"=w271) -> ("error out"=w282:errorcluster)  [unwired: 4 in, 1 out]
            n181 = call-poly "AO Update Channel.vi"("value"=w253, "channel (0)"="1", "device"=w254) -> ()
            n182 = call <vilib>:"Simple Error Handler.vi"("error in (no error)"=w282) -> ()  [unwired: 4 in, 5 out]
          }
        }
        n183 = stacked-sequence {
          tunnel: w105 -> [w119]
          frame #0 {
            w117 = T5 2 items=["ダイアログなし", "OKメッセージ", "継続か停止メッセージ", "OKメッセージ+警告", "継続/停止+警告"] ("ダイアログタイプ（OK msg:1）")
            n184 = local read "DeviceName"() -> (w123:tag)
            n185 = call "NIDAQ_AOInit(Single_update).vi"("DeviceName"=w123, "CH_A"=0, "CH_B"=1, "Single_point"=dbl[] [0.0, 0.0], "error in (no error)"=w119) -> ("error out"=w118:errorcluster)  [unwired: 10 in]
            n186 = call <vilib>:"Simple Error Handler.vi"("type of dialog (OK msg:1)"=w117, "error in (no error)"=w118) -> ()  [unwired: 3 in, 5 out]
          }
        }
        n187 = Array Max & Min(array=w113) -> (max index (indices)=w109:i32, min index (indices)=w111:i32)  [unwired: 2 out]
        n188 = property on="CZE" class="XYGraph (严格)"("Xスケール.表示形式:精度"=u8 1 ("X Precision"), "Xスケール.スケールフィット"=u8 1 ("X Scale Fit"), "アクティブカーソル"=u32 0 ("Active Cursor"), "カーソル.カーソルロックスタイル"=u32 1 ("Cursor Locked"), "カーソル.カーソル指標"=w109, "アクティブカーソル"=u32 1 ("Active Cursor"), "カーソル.カーソルロックスタイル"=u32 1 ("Cursor Locked"), "カーソル.カーソル指標"=w111) -> ()  [unwired: 2 in, 2 out]
      }
      frame 4 {
        # "store data"
        # "Returns Not A Path if Cancel"
        n189 = Unbundle(w348) -> ("all rows"=w346:dbl[], "all rows"=w347:dbl[])
        n190 = Build Array(w346, w347) -> (w345:dbl[][])
        n191 = Transpose 2D Array(2D array=w345) -> (transposed array=w358:dbl[][])
        n192 = Array To Spreadsheet String(array=w358, 3:"%.6f" ("format string")) -> (spreadsheet string=w352:string)  [unwired: 1 in]
        n193 = call <vilib>:"Open_Create_Replace File.vi"("pattern"="*.TXT", "prompt"="Save Data", "function (open:0)"=T4."create or replace") -> ("error out"=w353:errorcluster, "new file path"=w360:path, "refnum"=w354:refnum<file>)  [unwired: 5 in, 1 out]
        n194 = Not A Number/Path/Refnum?(number/path/refnum=w360) -> (NaN/Path/Refnum?=w364:bool)
        n195 = Write to Binary File(file (use dialog)=w354, data=w352, error in=w353, 5:FALSE ("配列または文字列サイズを先頭に追加?（T）")) -> (refnum out=w355:refnum<file>, error out=w356:errorcluster)  [unwired: 2 in, 1 out]
        n196 = Close File(refnum=w355, error in=w356) -> (error out=w357:errorcluster)  [unwired: 1 out]
        n197 = Select(t=i16 0, s=w364, f=i16 1) -> (s? t:f=w361:i16)
        n198 = call <vilib>:"Simple Error Handler.vi"("type of dialog (OK msg:1)"=w361, "error in (no error)"=w357) -> ()  [unwired: 3 in, 5 out]
      }
      frame 5 {
        # "only update XY graph\nif valid file name selected"
        # "CZE xy graph"
        # "Read data"
        n199 = case shown="假" "ケース定数\\n（詳細ヘルプを参照）" {
          frame False {
            # "Returns Not A Path if Cancel"
            n200 = call <vilib>:"Open_Create_Replace File.vi"("pattern"="*.TXT", "prompt"="Save EChem Data", "function (open:0)"=T4."open") -> ("error out"=w389:errorcluster, "new file path"=w395:path, "refnum"=w390:refnum<file>)  [unwired: 5 in, 1 out]
            n201 = Not A Number/Path/Refnum?(number/path/refnum=w395) -> (NaN/Path/Refnum?=w399:bool)
            n202 = Read from Binary File(5:4 ("byte stream type"), 8:w389, 11:w390) -> (0:w392:errorcluster, 3:w391:refnum<file>)  [unwired: 3 in, 2 out]
            n203 = Select(t=i16 0, s=w399, f=i16 1) -> (s? t:f=w396:i16)
            n204 = Close File(refnum=w391, error in=w392) -> (error out=w393:errorcluster)  [unwired: 1 out]
            n205 = call <vilib>:"Simple Error Handler.vi"("type of dialog (OK msg:1)"=w396, "error in (no error)"=w393) -> ()  [unwired: 3 in, 5 out]
          }
          frame True {
          }
        }
        n206 = call-poly <vilib>:"Read From Spreadsheet File.vi"("transpose (no:F)"=TRUE) -> ("all rows"=w373:dbl[][], "new file path (Not A Path if cancelled)"=w371:path)  [unwired: 6 in, 3 out]
        n207 = Not Equal?(x=path "", y=w371) -> (x != y?=w369:bool)
        n208 = property on="file name" class="Str"("表示"=w369) -> ()  [unwired: 2 in, 2 out]
        n209 = case shown="真" w369 {
          tunnel: w371 -> [_ w384]
          frame False {
          }
          frame True {
            n210 = Strip Path(path=w384) -> (name=→"file name":string)  [unwired: 1 out]
          }
        }
        n211 = Index Array(array=w373, index (row)=0) -> (element=w370:dbl[])  [unwired: 1 in]
        n212 = Index Array(array=w373, index (row)=1) -> (element=w377:dbl[])  [unwired: 1 in]
        n213 = Array Max & Min(array=w377) -> (max index (indices)=w376:i32, min index (indices)=w375:i32)  [unwired: 2 out]
        n214 = Bundle("all rows"=w370, "all rows"=w377) -> (w367:cluster{"all rows":dbl[], "all rows":dbl[]})  [unwired: 1 in]
        n215 = property on="CZE" class="XYGraph (严格)"("アクティブカーソル"=u32 0 ("Active Cursor"), "カーソル.カーソル指標"=w376, "アクティブカーソル"=u32 1 ("Active Cursor"), "カーソル.カーソル指標"=w375) -> ()  [unwired: 2 in, 2 out]
        n216 = Select(t=w367, s=w369, f=w366) -> (s? t:f=w368:cluster{"all rows":dbl[], "all rows":dbl[]})
        n217 = local write "CZE"(w368) -> ()
      }
    }
    n218 = Wait (ms)(milliseconds to wait=u32 50) -> ()  [unwired: 1 out]
  }
  n219 = local read "DeviceName"() -> (w1:tag)
  n220 = call "NIDAQ_AOInit(Single_update).vi"("DeviceName"=w1, "CH_A"=0, "CH_B"=1, "Single_point"=dbl[] [0.0, 0.0], "error in (no error)"=w2) -> ()  [unwired: 10 in, 1 out]
